vi "Batch Messaging.vi"() -> (3 "Pass?":bool)   [LabVIEW 2014]
uses:
  TestActor/TestActor.lvclass
  <vilib>/ActorFramework/LastAck/Last Ack.lvclass
  Increment Msg/Increment Msg.lvclass/Increment Msg.ctl
  <vilib>/ActorFramework/Message Queue/Message Queue.lvclass/Message Queue.ctl
  <vilib>/ActorFramework/Batch Msg/Batch Msg.lvclass/Batch Msg.ctl
  <vilib>/ActorFramework/Message Enqueuer/Message Enqueuer.lvclass/Message Enqueuer.ctl
  <vilib>/ActorFramework/Message Dequeuer/Message Dequeuer.lvclass/Message Dequeuer.ctl
  <vilib>/ActorFramework/LastAck/Last Ack.lvclass/Last Ack.ctl
  TestActor/TestActor.lvclass/TestActor.ctl
  <vilib>/ActorFramework/Message Enqueuer/Enqueue.vi
  <vilib>/ActorFramework/Message Priority Queue/Priority Dequeue.vi
  <vilib>/ActorFramework/Message Priority Queue/Priority Enqueue.vi
  Increment Msg/Increment Msg.lvclass
  <vilib>/ActorFramework/Batch Msg/Batch Msg.lvclass
  <vilib>/ActorFramework/Stop Msg/Stop Msg.lvclass
  <vilib>/ActorFramework/Actor/Actor.lvclass
  <vilib>/ActorFramework/Message Queue/Message Queue.lvclass
  <vilib>/ActorFramework/Message Dequeuer/Message Dequeuer.lvclass
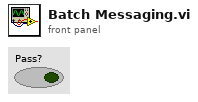
[diagram p1: front panel]
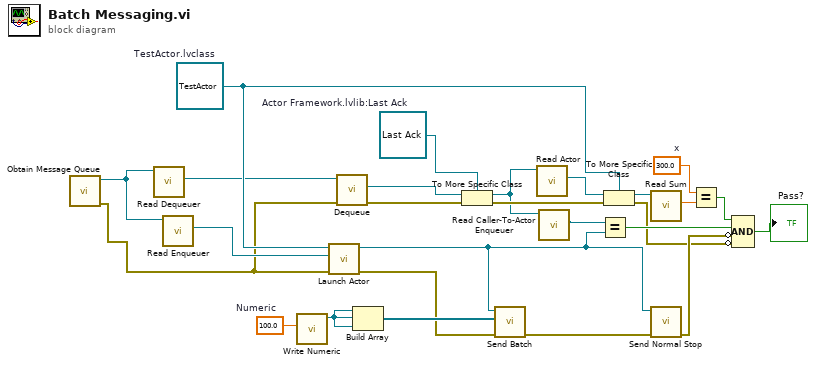
[diagram p0: block diagram]
diagram:
  w14 = 100.0  # Numeric
  w20 = 300.0  # x
  w26 = refnum<class "Last Ack.lvclass"> refnum  # Actor Framework.lvlib:Last Ack
  w23 = refnum<class "TestActor.lvclass"> refnum  # TestActor.lvclass
  n1 = call <vilib>:"Obtain Message Queue.vi"() -> ("error out"=w5:errorcluster, "Message Queue"=w8:refnum<class "Message Queue.lvclass">)  [unwired: 10 in]
  n2 = call <vilib>:"Read Dequeuer.vi"("Message Queue"=w8) -> ("Message Dequeuer"=w6:refnum<class "Message Dequeuer.lvclass">)  [unwired: 10 in]
  n3 = call <vilib>:"Read Enqueuer.vi"("Message Queue"=w8) -> ("Message Enqueuer"=w7:refnum<class "Message Enqueuer.lvclass">)  [unwired: 10 in]
  n4 = call "Write Numeric.vi"("Numeric"=w14) -> ("Increment Msg out"=w13:refnum<class "Increment Msg.lvclass">)  [unwired: 10 in]
  n5 = call <vilib>:"Launch Actor.vi"("error in (no error)"=w5, "Actor-to-Caller Enqueuer"=w7, "Actor"=w23) -> ("error out"=w10:errorcluster, "Caller-To-Actor Enqueuer"=w12:refnum<class "Message Enqueuer.lvclass">)  [unwired: 7 in]
  n6 = call <vilib>:"Dequeue.vi"("error in (no error)"=w5, "Message Dequeuer in"=w6) -> ("error out"=w4:errorcluster, "Message"=w3:refnum<class "Message.lvclass">)  [unwired: 5 in, 3 out]
  n7 = Build Array(w13, w13, w13) -> (w11:refnum<class "Increment Msg.lvclass">[])
  n8 = To More Specific Class(target class=w26, reference=w3, error in=w4) -> (specific class reference=w2:refnum<class "Last Ack.lvclass">, error out=w25:errorcluster)
  n9 = call <vilib>:"Send Batch.vi"("error in (no error)"=w10, "Messages Array"=w11, "Message Enqueuer"=w12) -> ("error out"=w9:errorcluster)  [unwired: 8 in]
  n10 = call <vilib>:"Read Actor.vi"("Last Ack"=w2) -> ("Actor"=w24:refnum<class "Actor.lvclass">)  [unwired: 10 in]
  n11 = call <vilib>:"Read Caller-To-Actor Enqueuer.vi"("Last Ack"=w2) -> ("Caller-to-Actor Enqueuer"=w1:refnum<class "Message Enqueuer.lvclass">)  [unwired: 10 in]
  n12 = Equal?(x=w1, y=w12) -> (x = y?=w18:bool)
  n13 = To More Specific Class(target class=w23, reference=w24, error in=w25) -> (specific class reference=w22:refnum<class "TestActor.lvclass">, error out=w15:errorcluster)
  n14 = call "Read Sum.vi"("TestActor in"=w22) -> ("Sum"=w21:dbl)  [unwired: 9 in, 1 out]
  n15 = call <vilib>:"Send Normal Stop.vi"("error in (no error)"=w9, "Message Enqueuer"=w12) -> ("error out"=w16:errorcluster)  [unwired: 9 in]
  n16 = Equal?(x=w20, y=w21) -> (x = y?=w19:bool)
  n17 = Compound Arithmetic op=AND(w19, w18, invert w16, invert w15) -> (→"Pass?":bool)
